vi "okCFrontPanelDevices Get Device Refnum.vi"(8 "Error In":errorcluster, 9 "Serial Number":string, 11 "okCFrontPanelDevices Refnum":refnum<k24>) -> (0 "Error Out":errorcluster, 1 "Device Refnum":refnum<k24>, 3 "okCFrontPanelDevices Refnum":refnum<k24>)   [LabVIEW 2021, in "okFrontPanelC#Wrapper.lvlib"]
uses:
  okFrontPanelC#Wrapper.lvlib
  D:/UCLA Thinkpad Google Drive/LabVIEW 2021 SP1/builds/SwissSPAD Live Distribution/Opal Kelly/C# Wrapper/v5.0.2/libFrontPanel-csharp.dll
  v5.0.2/libFrontPanel-csharp.dll
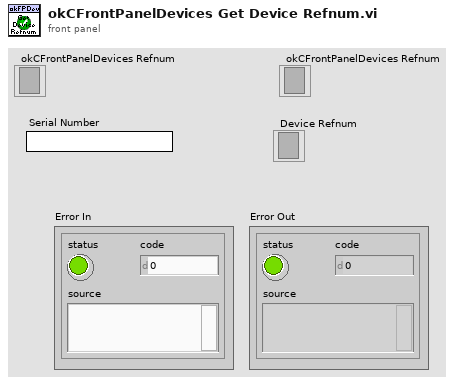
[diagram p1: front panel]
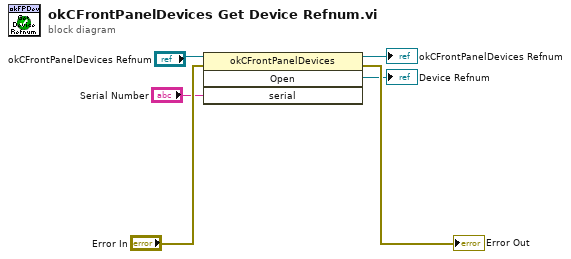
[diagram p0: block diagram]
diagram:
  n1 = invoke class="okCFrontPanelDevices" method="Open"(reference="okCFrontPanelDevices Refnum", error in="Error In", "serial"="Serial Number") -> (reference out=→"okCFrontPanelDevices Refnum":refnum<k24>, error out=→"Error Out":errorcluster, "Open"=→"Device Refnum":refnum<k24>)  [unwired: 1 in, 1 out]
